vi "PH_BL-Master.PC _getO2Conctr.vi"(0 "i ref in":refnum<vi>, 2 "O2 Instance":string="N/A", 3 "Concentration [%]":dbl, 4 "no link":bool, 5 "error in (no error)":errorcluster) -> (14 "i ref out":refnum<vi>, 19 "error out":errorcluster)   [LabVIEW 2014, in "PH_BL-Master.lvlib"]
doc: "This VI writes the incoming information to own attributes."
uses:
  PH_BL-Master.lvlib
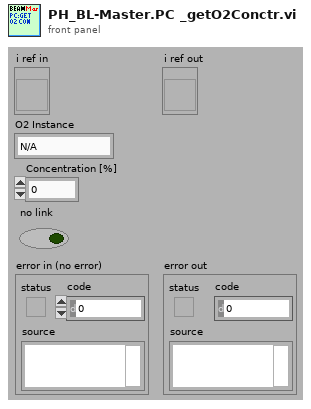
[diagram p1: front panel]
types:
  T1 = typedef "PH_BL-Master.lvlib/PH_BL-Master.i attribute.ctl" = cluster{"Remote controlled":bool, "Boolean Condition Service Subscriber":refnum<vi>[], "Picture Condition Service Subscriber":refnum<vi>[], "R2S":cluster{"GUI Ref":refnum<vi>, "State":bool}, "Vacua":cluster{"GUI Ref":refnum<vi>, "Limit":dbl, "Curr Value":dbl, "in range":bool}[], "O2 Inspection":cluster{"GUI Ref":refnum<vi>, "Concentration":dbl, "State":T2}[], "Boolean Status Service Subscriber":cluster{"GUI Ref":refnum<vi>, "Status":T2, "no Link?":bool, "Status Subscriber Class":T3}[], "Picture Status Service Subscriber":cluster{"GUI Ref":refnum<vi>, "Status":T2, "no Link?":bool, "Status Subscriber Class":T3}[], "6P 4Q Service Subscriber":cluster{"GUI Ref":refnum<vi>, "Selector":T4, "no Link?":bool}[], "Index of latest 6P 4Q changing Instance":i32, "Index of latest Picture Status changing Instance":i32, "Index of latest Boolean Status changing Instance":i32, "Vision ID on same Node":string, "Start Phase over?":bool, "GUI Ref Delete":refnum<vi>}
  T2 = typedef "PH_StatusHandler.lvlib/PH_StatusHandler.Status.ctl" = i16
  T3 = typedef "PH_BL-Master.lvlib/PH_BL-Master.Status Subscriber Class.ctl" = enum16{"unknown", "Switch", "BB", "6P Switch", "Switch GUI", "Switch and 6P State", "Force Sensor"}
  T4 = typedef "PH_4_Pos_Selector.lvlib/PH_4_Pos_Selector.Position Selector.ctl" = u16
  T5 = cluster{"GUI Ref":refnum<vi>, "Concentration":dbl, "State":T2}[]
  T6 = cluster{"GUI Ref":refnum<vi>, "Concentration":dbl, "State":T2}
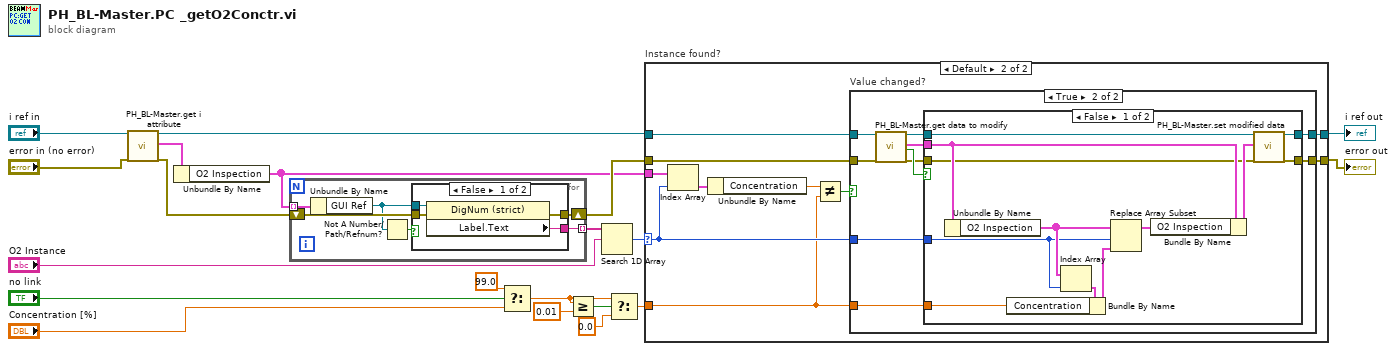
[diagram p0: block diagram]
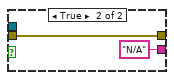
[diagram p5: hidden frame]
diagram:
  n1 = call "PH_BL-Master.get i attribute.vi"("i ref in"="i ref in", "error in (no error)"="error in (no error)") -> ("i ref out"=w16:refnum<vi>, "i attribute"=w15:T1, "error out"=w14:errorcluster)  [unwired: 15 in]
  n2 = Unbundle By Name(w15) -> ("O2 Inspection"=w2:T5)
  n3 = for {
    tunnel: w2 -> [w22] mode=indexing
    tunnel: [w26] -> w12 mode=indexing
    shift-right: [w24] -> w13
    shift-left: w14 -> [w25]
    n4 = Unbundle By Name(w22) -> ("GUI Ref"=w21:refnum<vi>)
    n5 = Not A Number/Path/Refnum?(number/path/refnum=w21) -> (NaN/Path/Refnum?=w23:bool)
    n6 = case shown="False" w23 {
      tunnel: w21 -> [w30 _]
      tunnel: [w29 "N/A" ("Label.Text")] -> w26
      tunnel: w25 -> [w28 w32]
      tunnel: [w27 w32] -> w24
      frame False {
        n7 = property class="DigNum (strict)"(reference=w30, error in=w28) -> (error out=w27:errorcluster, "Label.Text"=w29:string)  [unwired: 1 out]
      }
      frame True {
      }
    }
  }
  n8 = Select(t=99.0, s="no link", f="Concentration [%]") -> (s? t:f=w7:dbl)
  n9 = Greater Or Equal?(x=w7, y=0.01) -> (x >= y?=w8:bool)
  n10 = Search 1D Array(1D array=w12, element="O2 Instance") -> (index of element=w11:i32)  [unwired: 1 in]
  n11 = Select(t=w7, s=w8, f=0.0) -> (s? t:f=w3:dbl)
  n12 = case "Instance found?" shown="Default" w11 {
    selector: w11 -> [_ w39]
    tunnel: [w33 w44] -> w20
    tunnel: [w34 w43] -> w19
    tunnel: w3 -> [_ w36]
    tunnel: w16 -> [w34 w42]
    tunnel: w13 -> [w33 w41]
    tunnel: w2 -> [_ w40]
    frame -1 {
    }
    frame Default {
      n13 = Index Array(array=w40, index=w39) -> (element=w38:T6)
      n14 = Unbundle By Name(w38) -> ("Concentration"=w37:dbl)
      n15 = Not Equal?(x=w37, y=w36) -> (x != y?=w35:bool)
      n16 = case "Value changed?" shown="True" w35 {
        tunnel: [w45 w54] -> w44
        tunnel: [w46 w52] -> w43
        tunnel: w42 -> [w46 w50]
        tunnel: w41 -> [w45 w49]
        tunnel: w39 -> [_ w48]
        tunnel: w36 -> [_ w47]
        frame False {
        }
        frame True {
          n17 = call "PH_BL-Master.get data to modify.vi"("i ref in"=w50, "error in (no error)"=w49) -> ("i ref out"=w51:refnum<vi>, "i attribute"=w55:T1, "timed out"=w56:bool, "error out"=w53:errorcluster)  [unwired: 14 in]
          n18 = case shown="False" w56 {
            tunnel: w51 -> [w66 w70]
            tunnel: [w68 w70] -> w52
            tunnel: w53 -> [w58 w69]
            tunnel: [w67 w69] -> w54
            tunnel: w55 -> [w64 _]
            tunnel: w47 -> [w57 _]
            tunnel: w48 -> [w62 _]
            frame False {
              n19 = Unbundle By Name(w64) -> ("O2 Inspection"=w63:T5)
              n20 = Index Array(array=w63, index=w62) -> (element=w60:T6)
              n21 = Bundle By Name(cluster=w60, "Concentration"=w57) -> (w59:T6)
              n22 = Replace Array Subset(array=w63, new element=w59, index=w62) -> (w61:T5)
              n23 = Bundle By Name(cluster=w64, "O2 Inspection"=w61) -> (w65:T1)
              n24 = call "PH_BL-Master.set modified data.vi"("i ref in"=w66, "i attribute"=w65, "error in (no error)"=w58) -> ("i ref out"=w68:refnum<vi>, "error out"=w67:errorcluster)  [unwired: 15 in]
            }
            frame True {
            }
          }
        }
      }
    }
  }
  "error out" <- w20
  "i ref out" <- w19
